vi "cs_usb_open.vi"(2 "error in":errorcluster, 3 "sFileName":string="\\\\.\\EzUsb-0") -> (0 "error out":errorcluster={"status"=FALSE, "code"=0, "source"="fertig"}, 1 "handle":i32=1)   [LabVIEW 2017]
uses:
  kernel32.dll
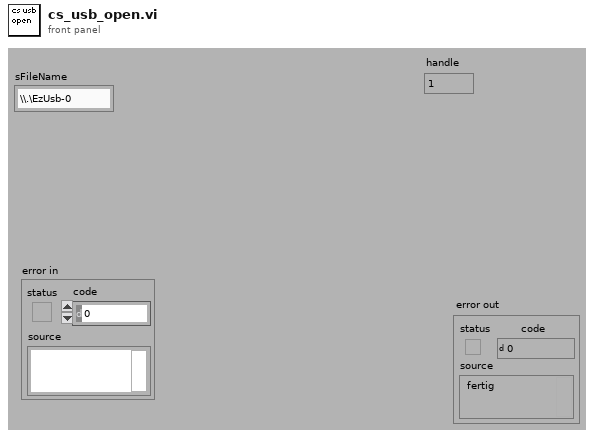
[diagram p1: front panel]
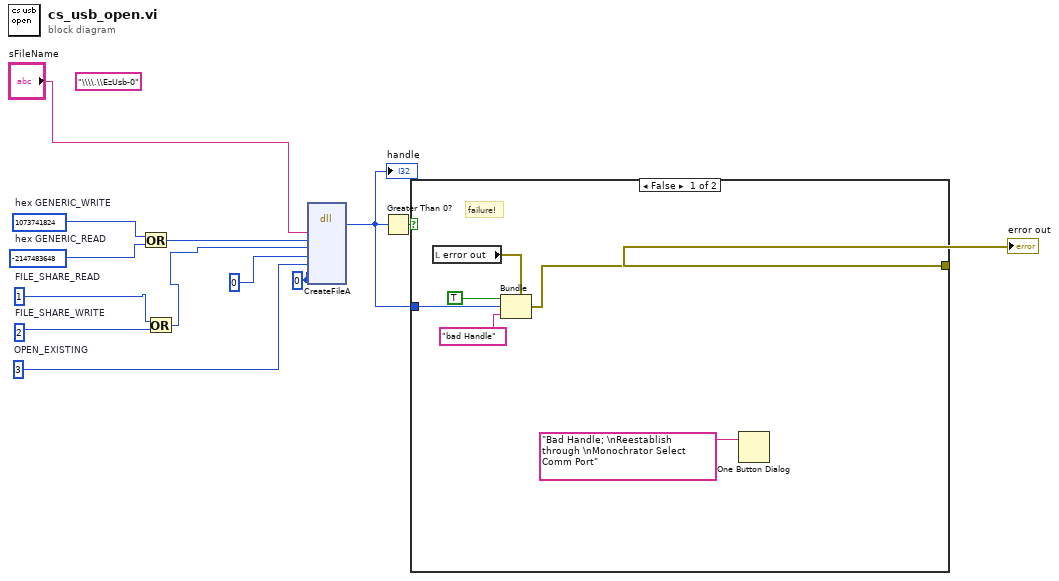
[diagram p0: block diagram]
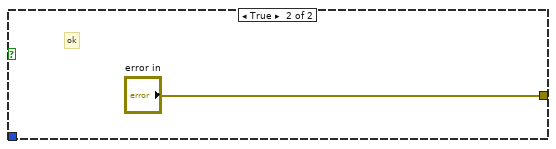
[diagram p2: hidden frame]
diagram:
  w9 = 3  # OPEN_EXISTING
  w4 = 2  # FILE_SHARE_WRITE
  w5 = 1  # FILE_SHARE_READ
  w12 = -2147483648  # hex GENERIC_READ
  w11 = 1073741824  # hex GENERIC_WRITE
  w13 = 0 ("null1")
  (unwired) "\\\\.\\EzUsb-0" ("sFileName")
  n1 = Or(x=w11, y=w12) -> (x .or. y?=w10:i32)
  n2 = Or(x=w5, y=w4) -> (x .or. y?=w6:i32)
  n3 = dll-call lib="kernel32.dll" fn="CreateFileA" label="CreateFile"("sFileName"="sFileName", "genericR_W"=w10, "fileshareR_W"=w6, "security"=0, "open_exist"=w9, "null1"=w13, "null2"=w13) -> ("handle"=w3:i32)  [unwired: 10 in, 2 out]
  "handle" <- w3
  n4 = Greater Than 0?(x=w3) -> (x > 0?=w8:bool)
  n5 = case shown="False" w8 {
    tunnel: w3 -> [w17 _]
    tunnel: [w15 "error in"] -> w2
    frame False {
      # "failure!"
      n6 = local read "error out"() -> (w16:errorcluster)
      n7 = Bundle(cluster=w16, "status"=TRUE, "code"=w17, "source"="bad Handle") -> (w15:errorcluster)
      n8 = One Button Dialog(message="Bad Handle; \nReestablish through \nMonochrator Select Comm Port") -> ()  [unwired: 1 in, 1 out]
    }
    frame True {
      # "ok"
    }
  }
  "error out" <- w2
